vi "part2Tx.vi"() -> ()   [LabVIEW 2013]
uses:
  <instrlib>/niUSRP/niUSRP Write Tx Data (CDB).vi
panel:
  in  "end of data?":bool
  out "coerced gain":dbl format="%#_6f"
  out "coerced carrier frequency":dbl=100000.0 format="%#_6p"
  out "coerced IQ rate":dbl=100000.0 format="%#_6p"
  out "error out":errorcluster
  in  "active antenna":string
  in  "carrier frequency":dbl=100000.0 format="%#_6p"
  in  "gain":dbl format="%#_6f"
  in  "IQ rate":dbl=100000.0 format="%#_6p"
  in  "device names":refnum<k15>
  in  "dimension size":i32
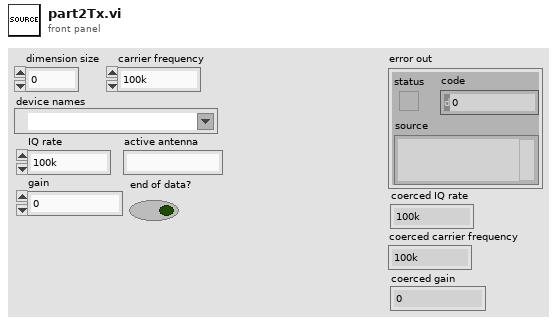
[diagram p1: front panel]
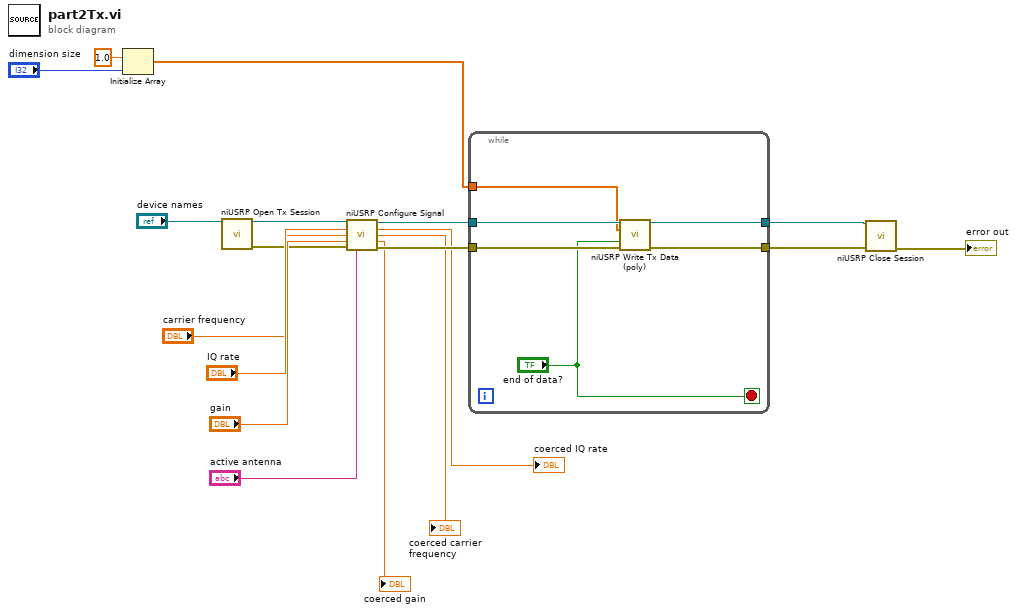
[diagram p0: block diagram]
diagram:
  n1 = Initialize Array(1.0 ("element"), "dimension size") -> (w2:dbl[])
  n2 = call <instrlib>:"niUSRP Open Tx Session.vi"("device names"="device names") -> ("session handle out"=w15:refnum<k15>, "error out"=w11:errorcluster)  [unwired: 13 in]
  n3 = call <instrlib>:"niUSRP Configure Signal.vi"("session handle"=w15, "IQ rate"="IQ rate", "carrier frequency"="carrier frequency", "gain"="gain", "error in (no error)"=w11, "active antenna"="active antenna") -> ("session handle out"=w3:refnum<k15>, "coerced IQ rate"=→"coerced IQ rate":dbl, "coerced carrier frequency"=→"coerced carrier frequency":dbl, "coerced gain"=→"coerced gain":dbl, "error out"=w9:errorcluster)  [unwired: 5 in]
  n4 = while {
    tunnel: w9 -> [w24]
    tunnel: [w23] -> w8
    tunnel: w3 -> [w21]
    tunnel: w2 -> [w20]
    tunnel: [w19] -> w1
    stop <- "end of data?" stop-if-true
    n5 = call-poly <instrlib>:"niUSRP Write Tx Data (poly).vi"("session handle"=w21, "data"=w20, "end of data?"="end of data?", "error in (no error)"=w24) -> ("session handle out"=w19:refnum<k15>, "error out"=w23:errorcluster)  [unwired: 10 in]
  }
  n6 = call <instrlib>:"niUSRP Close Session.vi"("session handle"=w1, "error in (no error)"=w8) -> ("error out"=→"error out":errorcluster)  [unwired: 13 in]
